vi "convertUDPMessage.vi"(8 "error in (no error)":errorcluster, 9 "message":string, 10 "user event out":refnum<user-event>) -> (0 "error out":errorcluster)   [LabVIEW 2011, in "Tools.lvlib" / "Imaging.lvlib" / "ImageAnalyser.lvclass"]
uses:
  ImageAnalyser.lvclass
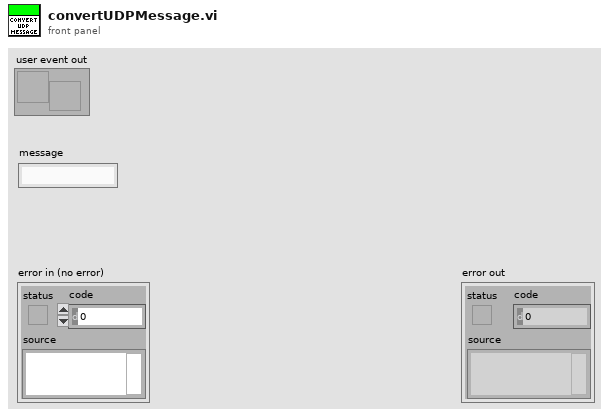
[diagram p1: front panel]
types:
  T1 = cluster{"cameraType":string, "imageName":string, "saved":string, "analysisType":string, "I16bit image data":u16[][], "path":path}
  T2 = typedef "Image Type" = u32
  T3 = typedef "IMAQ Image.ctl" = refnum<image>
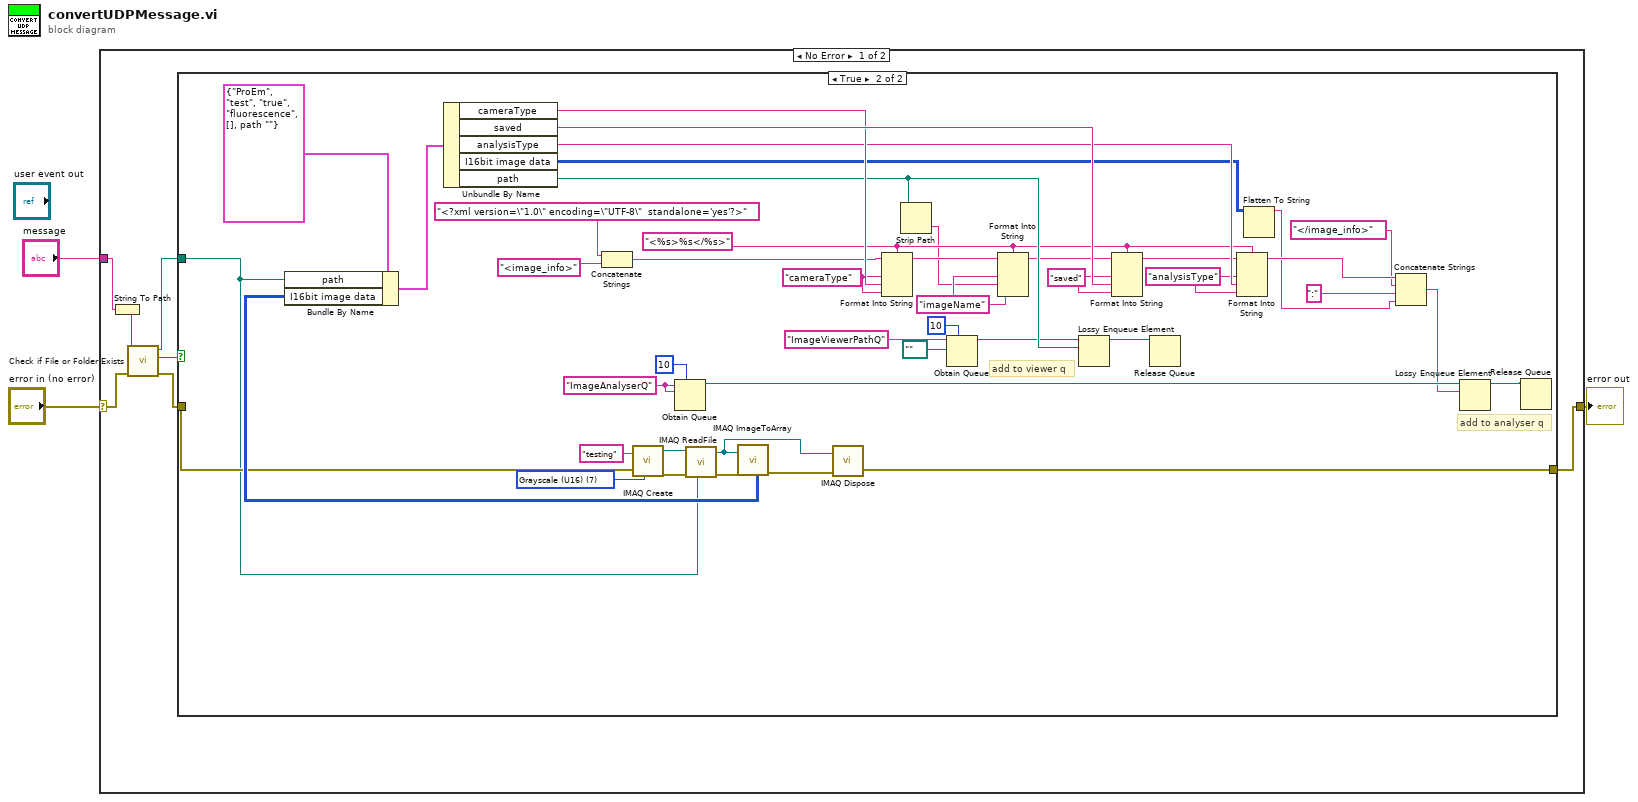
[diagram p0: block diagram]
diagram:
  n1 = case shown="No Error" "error in (no error)" {
    selector: "error in (no error)" -> [w9 w56]
    tunnel: [w10 w56] -> w2
    tunnel: "message" -> [w8 _]
    frame No Error {
      n2 = String To Path(string=w8) -> (path=w5:path)
      n3 = call <vilib>:"Check if File or Folder Exists.vi"("error in (no error)"=w9, "path"=w5) -> ("error out"=w7:errorcluster, "file or folder exists?"=w6:bool, "dup path"=w4:path)  [unwired: 7 in]
      n4 = case shown="True" w6 {
        tunnel: w7 -> [w11 w14]
        tunnel: [w11 w13] -> w10
        tunnel: w4 -> [_ w12]
        frame False {
        }
        frame True {
          w22 = T2 7 items=["Grayscale (U8)", "Grayscale (I16)", "Grayscale (SGL)", "Complex (CSG)", "RGB (U32)", "HSL (U32)", "RGB (U64)", "Grayscale (U16)"] ("Image Type")
          w41 = "analysisType"
          w39 = "saved"
          w35 = "imageName" ("Key")
          w34 = "cameraType"
          w46 = "ImageAnalyserQ"
          w47 = "<%s>%s</%s>"
          # "add to analyser q"
          # "add to viewer q"
          n5 = Concatenate Strings("<?xml version=\"1.0\" encoding=\"UTF-8\"  standalone='yes'?>", "<image_info>") -> (w48:string)
          n6 = call "IMAQ Create"("Image Name"="testing", "Image Type"=w22, "error in (no error)"=w14) -> ("New Image"=w21:T3, "error out"=w20:errorcluster)  [unwired: 2 in]
          n7 = Obtain Queue(max queue size (-1, unlimited)=10, name (unnamed)=w46, element data type=w46) -> (queue out=w44:refnum<queue>)  [unwired: 2 in, 2 out]
          n8 = call "IMAQ ReadFile"("File Path"=w12, "error in (no error)"=w20, "Image"=w21) -> ("error out"=w19:errorcluster, "Image Out"=w16:T3)  [unwired: 4 in, 3 out]
          n9 = call "IMAQ ImageToArray"("error in (no error)"=w19, "Image"=w16) -> ("Image Pixels (U16)"=w18:u16[][], "error out"=w17:errorcluster)  [unwired: 2 in, 3 out]
          n10 = Bundle By Name(cluster=T1 {"cameraType"="ProEm", "imageName"="test", "saved"="true", "analysisType"="fluorescence", "I16bit image data"=[], "path"=path ""} ("input cluster"), "path"=w12, "I16bit image data"=w18) -> (w24:T1)
          n11 = Unbundle By Name(w24) -> ("cameraType"=w54:string, "saved"=w55:string, "analysisType"=w53:string, "I16bit image data"=w52:u16[][], "path"=w51:path)
          n12 = call "IMAQ Dispose"("Image"=w16, "error in (no error)"=w17) -> ("error out"=w13:errorcluster)  [unwired: 4 in]
          n13 = Format Into String(format string=w47, initial string=w48, w34, w54, w34) -> (resulting string=w37:string)  [unwired: 1 in, 1 out]
          n14 = Strip Path(path=w51) -> (name=w33:string)  [unwired: 1 out]
          n15 = Obtain Queue(max queue size (-1, unlimited)=10, name (unnamed)="ImageViewerPathQ", element data type=path "") -> (queue out=w28:refnum<queue>)  [unwired: 2 in, 2 out]
          n16 = Format Into String(format string=w47, initial string=w37, w35, w33, w35) -> (resulting string=w38:string)  [unwired: 1 in, 1 out]
          n17 = Lossy Enqueue Element(queue=w28, element=w51) -> (queue out=w27:refnum<queue>)  [unwired: 1 in, 3 out]
          n18 = Format Into String(format string=w47, initial string=w38, w39, w55, w39) -> (resulting string=w42:string)  [unwired: 1 in, 1 out]
          n19 = Release Queue(queue=w27) -> ()  [unwired: 2 in, 3 out]
          n20 = Format Into String(format string=w47, initial string=w42, w41, w53, w41) -> (resulting string=w43:string)  [unwired: 1 in, 1 out]
          n21 = Flatten To String(anything=w52) -> (data string=w32:string)  [unwired: 3 in, 2 out]
          n22 = Concatenate Strings(w43, "</image_info>", ":", w32) -> (w15:string)
          n23 = Lossy Enqueue Element(queue=w44, element=w15) -> (queue out=w26:refnum<queue>)  [unwired: 1 in, 3 out]
          n24 = Release Queue(queue=w26) -> ()  [unwired: 2 in, 3 out]
        }
      }
    }
    frame Error {
    }
  }
  "error out" <- w2
